vi "Write Async Message Execution Status Map.vi"(8 "error in (no error)":errorcluster, 10 "Async Message Execution Status Map":T1, 11 "Async Methods Actor in":refnum<class "Async Methods Actor.lvclass">) -> (0 "error out":errorcluster, 3 "Async Methods Actor out":refnum<class "Async Methods Actor.lvclass">)   [LabVIEW 2021, in "Async Methods Actor.lvlib" / "Async Methods Actor.lvclass"]
uses:
  Async Methods Actor.lvclass
  Async Message Execution Status Map.ctl
  Async Message Execution Status.ctl
  Async Methods Running.ctl
  Async Methods Actor.lvclass/Async Methods Actor.ctl
  3adbf29e-89d7-4ecb-a2bd-8a8b89d527f8.vi
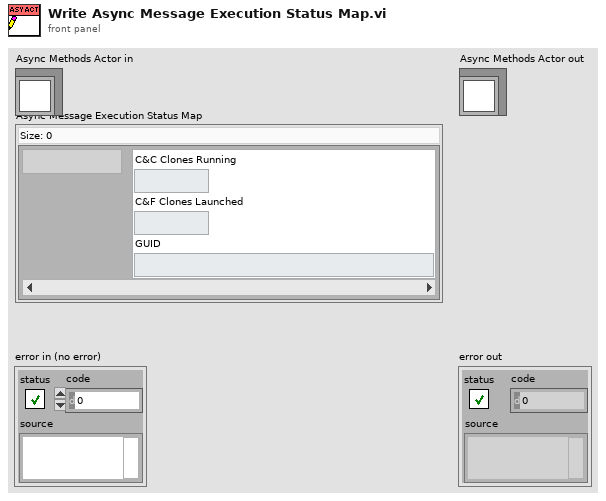
[diagram p1: front panel]
types:
  T1 = typedef "Async Methods Actor.lvlib/Async Methods Actor.lvclass/Async Message Execution Status Map.ctl" = map{string, T2}
  T2 = typedef "Async Methods Actor.lvlib/Async Methods Actor.lvclass/Async Message Execution Status.ctl" = cluster{"C&C Clones Running":u32, "C&F Clones Launched":u32, "GUID":string}
  T3 = typedef "Async Methods Actor.lvlib/Async Methods Actor.lvclass/Async Methods Running.ctl" = cluster{"Async Messages":string[], "C&C Running":u32[], "C&F Launched":u32[]}
  T4 = typedef "Async Methods Actor.lvlib/Async Methods Actor.lvclass/Running Methods Communication.ctl" = enum16{"None", "Notifier", "Event"}
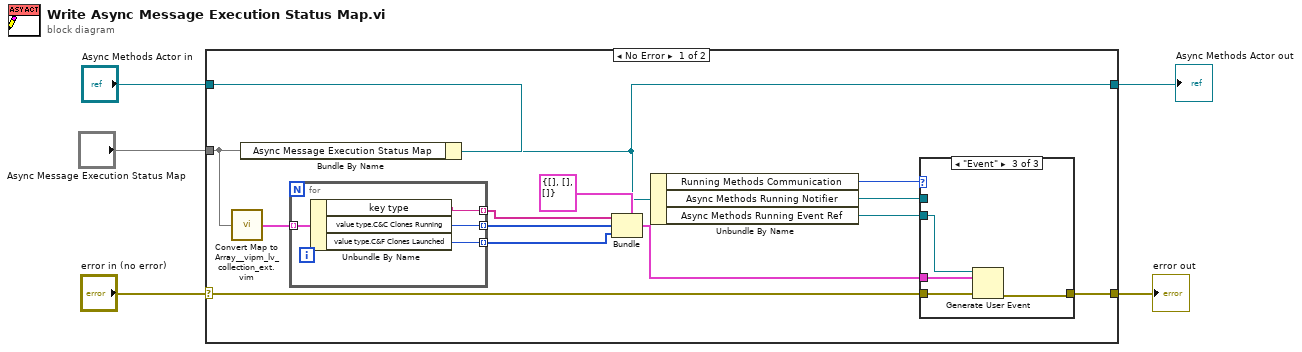
[diagram p0: block diagram]
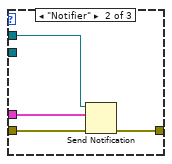
[diagram p3: hidden frame]
diagram:
  n1 = case shown="No Error" "error in (no error)" {
    selector: "error in (no error)" -> [w18 w33]
    tunnel: [w17 w33] -> w4
    tunnel: [w11 w34] -> w1
    tunnel: "Async Methods Actor in" -> [w19 w34]
    tunnel: "Async Message Execution Status Map" -> [w15 _]
    frame No Error {
      n2 = call "Convert Map to Array__vipm_lv_collection_ext.vim"("map"=w15) -> ("array"=w16:cluster{"key type":string, "value type":T2}[])  [unwired: 12 in, 2 out]
      n3 = Bundle By Name(cluster=w19, "Async Message Execution Status Map"=w15) -> (w11:refnum<class "Async Methods Actor.lvclass">)
      n4 = for {
        tunnel: w16 -> [w32] mode=indexing
        tunnel: [w31] -> w7 mode=indexing
        tunnel: [w30] -> w6 mode=indexing
        tunnel: [w29] -> w13 mode=indexing
        n5 = Unbundle By Name(w32) -> ("key type"=w29:string, "value type.C&C Clones Running"=w31:u32, "value type.C&F Clones Launched"=w30:u32)
      }
      n6 = Bundle(cluster=T3 {"Async Messages"=[], "C&C Running"=[], "C&F Launched"=[]} ("Async Methods Running"), "Async Messages"=w13, "C&C Running"=w7, "C&F Launched"=w6) -> (w12:T3)
      n7 = Unbundle By Name(w11) -> ("Running Methods Communication"=w9:T4, "Async Methods Running Notifier"=w10:refnum<notifier>, "Async Methods Running Event Ref"=w8:refnum<user-event>)
      n8 = case shown="\"Event\"" w9 {
        tunnel: w18 -> [w20 w24 w28]
        tunnel: [w20 w23 w27] -> w17
        tunnel: w12 -> [_ w22 w25]
        tunnel: w10 -> [_ w21 _]
        tunnel: w8 -> [_ _ w26]
        frame "None" {
        }
        frame "Notifier" {
          n9 = Send Notification(notification=w22, notifier=w21, error in (no error)=w24) -> (error out=w23:errorcluster)  [unwired: 1 out]
        }
        frame "Event" {
          n10 = Generate User Event(user event=w26, event data cluster=w25, error in=w28) -> (error out=w27:errorcluster)  [unwired: 1 in, 1 out]
        }
      }
    }
    frame Error {
    }
  }
  "error out" <- w4
  "Async Methods Actor out" <- w1
